vi "NET-RX TCP Service.vi"() -> ()   [LabVIEW 2014, in "GenNet-Server.lvlib"]
uses:
  GenNet-Server.lvlib
  DQMH-GenNet Message Queue.lvclass
  Stop Argument--cluster.ctl
  <vilib>/Delacor/Delacor QMH/Libraries/Message Queue_class/Delacor_lib_QMH_Message Queue.lvclass/Delacor_lib_QMH_Message Queue.ctl
  <vilib>/Delacor/Delacor QMH/Libraries/Message Queue_class/Delacor_lib_QMH_Enqueue Message (Single).vi
  GenNet Version-Safe Unflatten Variant.vi
  <vilib>/Delacor/Delacor QMH/Libraries/Message Queue_class/Delacor_lib_QMH_Message Queue.lvclass
  hse-gennet.lvlib
panel:
  in  "Notifier Timeout":i32=5000
  in  "Stop Module":refnum<user-event>
  in  "Module ID":i32=-1
  in  "Caller MsgQ":refnum<class "DQMH-GenNet Message Queue.lvclass">
  in  "Connection ID":refnum<k5>
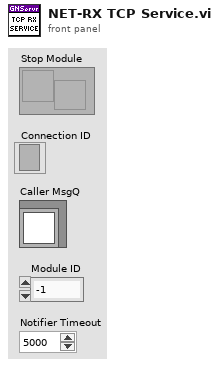
[diagram p1: front panel]
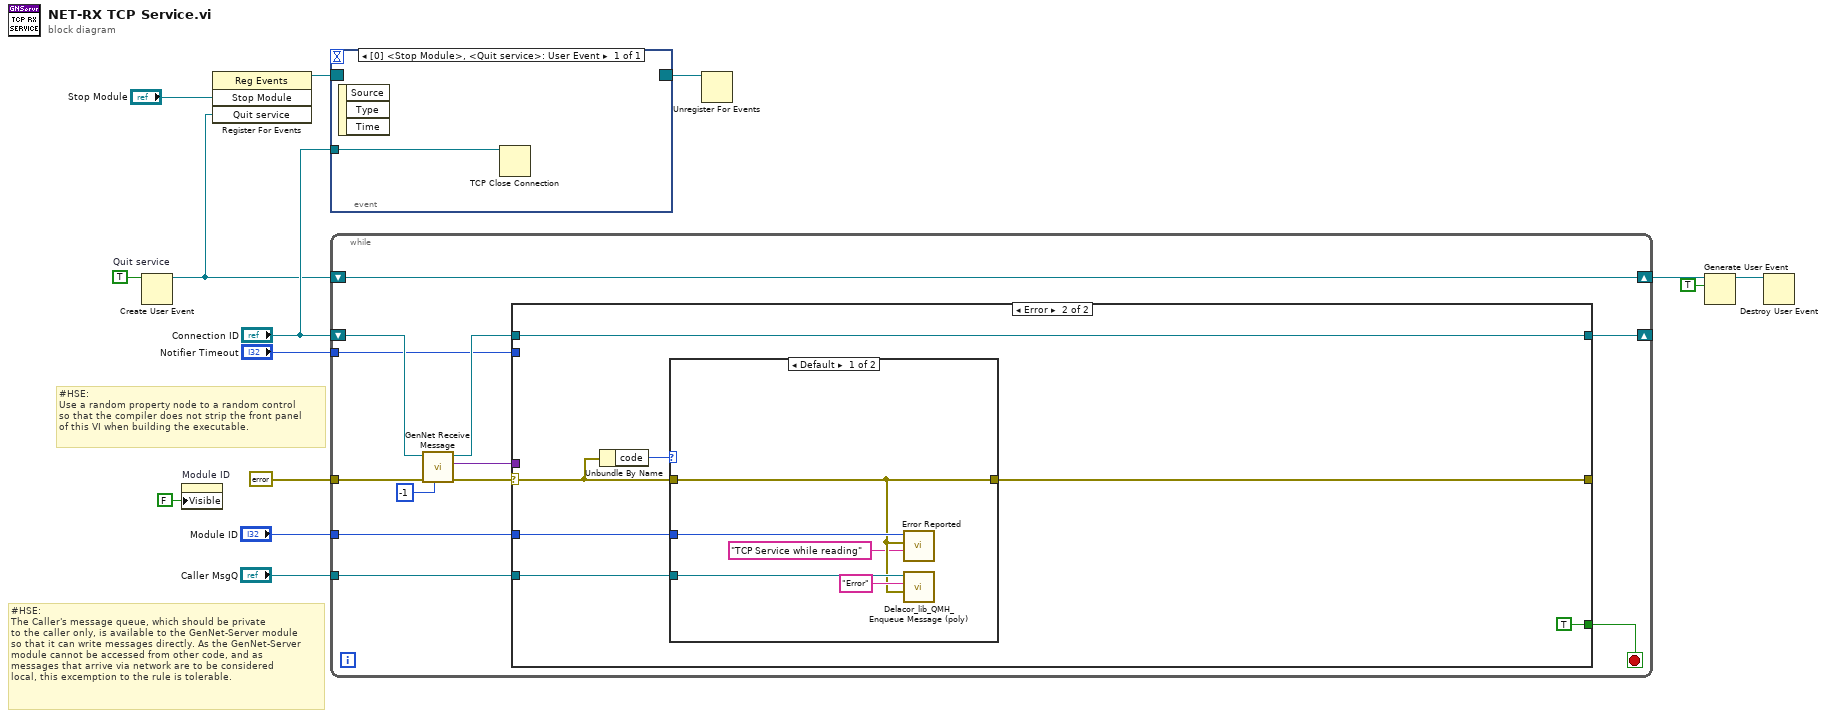
[diagram p0: block diagram]
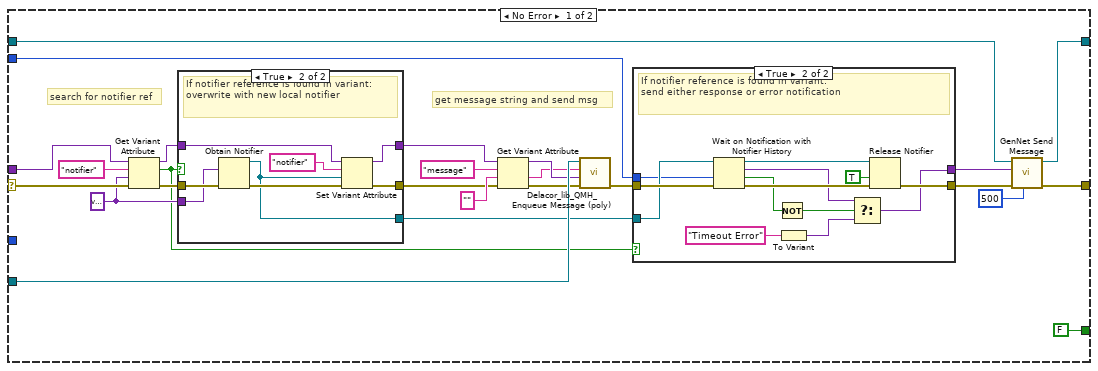
[diagram p2: hidden frame]
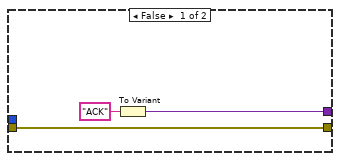
[diagram p3: hidden frame]
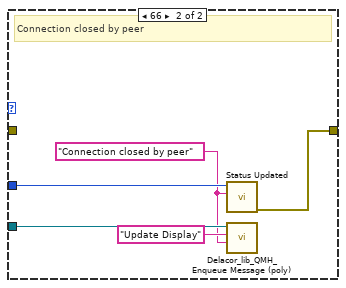
[diagram p5: hidden frame]
diagram:
  w11 = TRUE  # Quit service
  # "#HSE: \nUse a random property node to a random control \nso that the compiler does not strip the front panel \nof this VI when building the executable."
  # "#HSE: \nThe Caller's message queue, which should be private \nto the caller only, is available to the GenNet-Server module \nso that it can write messages directly. As the GenNet-Server\nmodule cannot be accessed from other code, and as \nmessages that arrive via network are to be considered \nlocal, this excemption to the rule is tolerable."
  n1 = Create User Event(user event datatype=w11) -> (user event=w10:refnum<user-event>)  [unwired: 1 in, 1 out]
  n2 = property on="Module ID" class="DigNum (strict)"("Visible"=FALSE) -> ()  [unwired: 2 in, 2 out]
  n3 = register-events("Stop Module", w10) -> (reference out=w13:refnum<event-registration>)  [unwired: 2 in, 1 out]
  n4 = event shown="[0] <Stop Module>, <Quit service>: User Event" {
    selector: w13 -> [_]
    dyn-events: [_] -> w6
    timeout: _ -> [_]
    tunnel: "Connection ID" -> [w15]
    event User Event {
      n5 = event-data() -> ()  [unwired: 1 in, 3 out]
      n6 = TCP Close Connection(connection ID=w15) -> ()  [unwired: 2 in, 2 out]
    }
  }
  n7 = while {
    shift-right: [w27] -> _
    shift-left: "Connection ID" -> [w19]
    tunnel: errorcluster {"status"=FALSE, "code"=0, "source"=""} ("error out") -> [w21]
    shift-right: [w26] -> w9
    shift-left: w10 -> [w26]
    tunnel: "Module ID" -> [w24]
    tunnel: "Caller MsgQ" -> [w23]
    tunnel: "Notifier Timeout" -> [w16]
    stop <- w25 stop-if-true
    n8 = call "GenNet Receive Message.vi"("timeout [ms]"=-1, "error in (no error)"=w21, "TCP Network Connection in"=w19) -> ("error out"=w20:errorcluster, "Message Data"=w17:variant, "TCP Network Connection out"=w18:refnum<k5>)  [unwired: 6 in]
    n9 = case shown="Error" w20 {
      selector: w20 -> [w49 w82]
      tunnel: w18 -> [w51 w80]
      tunnel: [w50 w80] -> w27
      tunnel: [FALSE TRUE] -> w25
      tunnel: w24 -> [_ w81]
      tunnel: w23 -> [w46 w83]
      tunnel: w17 -> [w48 _]
      tunnel: [w30 w79] -> _
      tunnel: w16 -> [w29 _]
      frame No Error {
        w42 = variant ("Message Data")
        # "get message string and send msg"
        # "search for notifier ref"
        n10 = Get Variant Attribute(Variant=w48, name="notifier", default value (empty Variant)=w42, error in=w49) -> (duplicate Variant=w44:variant, found=w35:bool, error out=w43:errorcluster)  [unwired: 1 out]
        n11 = case shown="True" w35 {
          tunnel: w44 -> [w70 w75]
          tunnel: w42 -> [_ w77]
          tunnel: w43 -> [w69 w78]
          tunnel: [w70 w73] -> w38
          tunnel: [w69 w72] -> w39
          tunnel: [_ w71] -> w31
          frame False {
          }
          frame True {
            # "If notifier reference is found in variant:\noverwrite with new local notifier"
            n12 = Obtain Notifier(notification data type=w77, error in (no error)=w78) -> (notifier out=w71:refnum<notifier>, error out=w76:errorcluster)  [unwired: 2 in, 1 out]
            n13 = Set Variant Attribute(Variant=w75, name="notifier", value=w71, error in=w76) -> (Variant out=w73:variant, error out=w72:errorcluster)  [unwired: 1 out]
          }
        }
        n14 = Get Variant Attribute(Variant=w38, name="message", default value (empty Variant)="", error in=w39) -> (duplicate Variant=w37:variant, value=w28:string, error out=w36:errorcluster)  [unwired: 1 out]
        n15 = call-poly <vilib>:"Delacor_lib_QMH_Enqueue Message (poly).vi"("error in (no error)"=w36, "Message Data"=w37, "Message"=w28, "Message Queue in"=w46) -> ("error out"=w34:errorcluster)  [unwired: 6 in, 1 out]
        n16 = case shown="True" w35 {
          tunnel: w34 -> [w55 w68]
          tunnel: [w55 w64] -> w33
          tunnel: [w54 w60] -> w32
          tunnel: w31 -> [_ w67]
          tunnel: w29 -> [_ w56]
          frame False {
            n17 = To Variant(anything="ACK") -> (Variant=w54:variant)
          }
          frame True {
            # "If notifier reference is found in variant:\nsend either response or error notification"
            n18 = Wait on Notification with Notifier History(0:w67, 2:w56, 3:w68) -> (8:w66:refnum<notifier>, 9:w61:variant, 10:w62:bool, 11:w65:errorcluster)  [unwired: 1 in]
            n19 = Not(x=w62) -> (.not. x?=w57:bool)
            n20 = To Variant(anything="Timeout Error") -> (Variant=w58:variant)
            n21 = Select(t=w61, s=w57, f=w58) -> (s? t:f=w60:variant)
            n22 = Release Notifier(notifier=w66, force destroy? (F)=TRUE, error in (no error)=w65) -> (error out=w64:errorcluster)  [unwired: 2 out]
          }
        }
        n23 = call "GenNet Send Message.vi"("timeout [ms]"=500, "error in (no error)"=w33, "Message Data"=w32, "TCP Network Connection in"=w51) -> ("error out"=w30:errorcluster, "TCP Network Connection out"=w50:refnum<k5>)  [unwired: 6 in]
      }
      frame Error {
        n24 = Unbundle By Name(w82) -> ("code"=w84:i32)
        n25 = case shown="Default" w84 {
          tunnel: w83 -> [w89 w94]
          tunnel: w82 -> [w87 _]
          tunnel: w81 -> [w88 w93]
          tunnel: [w87 w92] -> w79
          frame Default {
            n26 = call "Error Reported.vi"("Additional Information"="TCP Service while reading", "Error"=w87, "Module ID"=w88) -> ()  [unwired: 8 in, 1 out]
            n27 = call-poly <vilib>:"Delacor_lib_QMH_Enqueue Message (poly).vi"("Message Data"=w87, "Message"="Error", "Message Queue in"=w89) -> ()  [unwired: 7 in, 2 out]
          }
          frame 66 {
            w91 = "Connection closed by peer" ("format string")
            # "Connection closed by peer"
            n28 = call "Status Updated.vi"("Status"=w91, "Module ID"=w93) -> ("error out"=w92:errorcluster)  [unwired: 9 in]
            n29 = call-poly <vilib>:"Delacor_lib_QMH_Enqueue Message (poly).vi"("Message Data"=w91, "Message"="Update Display", "Message Queue in"=w94) -> ()  [unwired: 7 in, 2 out]
          }
        }
      }
    }
  }
  n30 = Unregister For Events(event registration refnum=w6) -> ()  [unwired: 1 in, 1 out]
  n31 = Generate User Event(user event=w9, event data cluster=TRUE ("event data")) -> (user event out=w7:refnum<user-event>)  [unwired: 2 in, 1 out]
  n32 = Destroy User Event(user event=w7) -> ()  [unwired: 1 in, 1 out]
